vi "Read Ctrl_.vi"(8 "error in (no error)":errorcluster, 11 "Keyboard Macro in":refnum<class "Keyboard Macro.lvclass">) -> (0 "error out":errorcluster, 2 "Ctrl?":bool, 3 "Keyboard Macro out":refnum<class "Keyboard Macro.lvclass">)   [LabVIEW 2020, in "MacroAssert.lvlib" / "Keyboard Macro.lvclass"]
uses:
  Keyboard Macro.lvclass
  Keyboard Macro.lvclass/Keyboard Macro.ctl
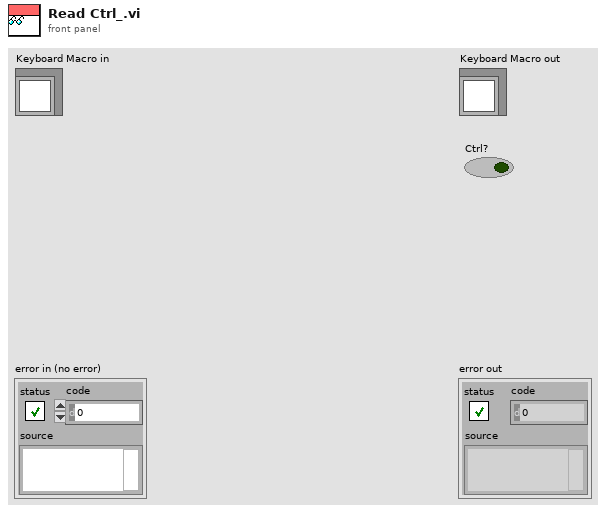
[diagram p1: front panel]
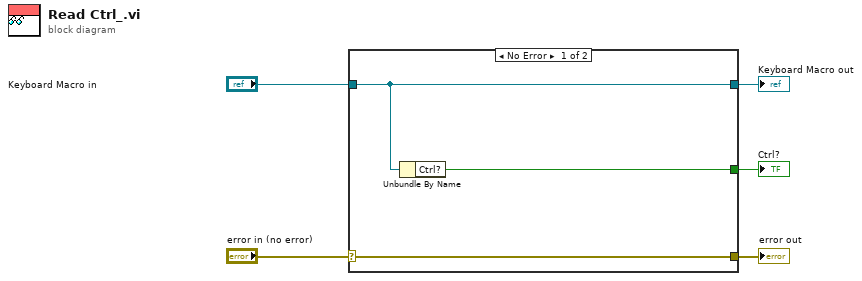
[diagram p0: block diagram]
diagram:
  n1 = case shown="No Error" "error in (no error)" {
    selector: "error in (no error)" -> [w8 w9]
    tunnel: [w8 w9] -> w4
    tunnel: [w7 w10] -> w2
    tunnel: "Keyboard Macro in" -> [w7 w10]
    tunnel: [w6 _] -> w1
    frame No Error {
      n2 = Unbundle By Name(w7) -> ("Ctrl?"=w6:bool)
    }
    frame Error {
    }
  }
  "error out" <- w4
  "Keyboard Macro out" <- w2
  "Ctrl?" <- w1
